vi "ELAPSED TIMER VI FOR Sway Loop Connection.vi"(8 "error in":errorcluster, 9 "TARGET":dbl, 10 "RESET":bool, 11 "PAUSE":bool) -> (0 "error out":errorcluster, 1 "ELAPSED INDICATION":bool, 2 "ELAPSED TIMER":dbl)   [LabVIEW 2025]
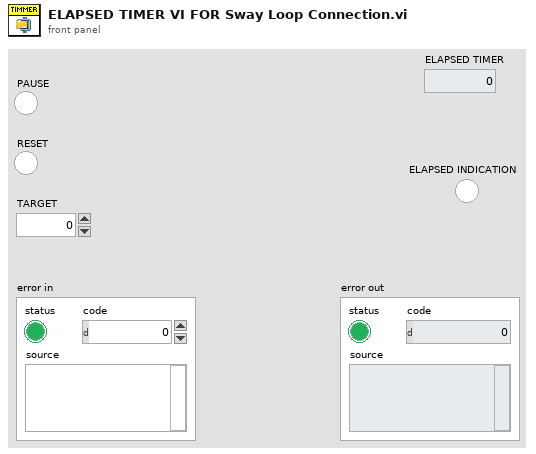
[diagram p1: front panel]
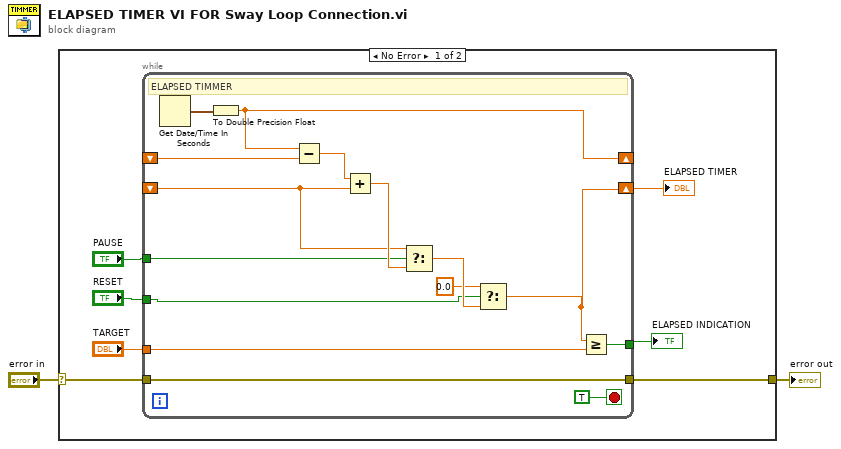
[diagram p0: block diagram]
diagram:
  n1 = case shown="No Error" "error in" {
    selector: "error in" -> [w4 _]
    tunnel: [w3 _] -> w1
    frame No Error {
      n2 = while {
        shift-right: [w21] -> _
        shift-left: _ -> [w22]
        shift-right: [w13] -> w6
        shift-left: _ -> [w18]
        tunnel: "PAUSE" -> [w17]
        tunnel: "RESET" -> [w14]
        tunnel: "TARGET" -> [w12]
        tunnel: [w11] -> w5
        tunnel: w4 -> [w10]
        tunnel: [w10] -> w3
        stop <- TRUE stop-if-true
        # "ELAPSED TIMMER"
        n3 = Get Date/Time In Seconds() -> (seconds since 1Jan1904=w23:timestamp)
        n4 = To Double Precision Float(number=w23) -> (double precision float=w21:dbl)
        n5 = Subtract(x=w21, y=w22) -> (x-y=w20:dbl)
        n6 = Add(x=w20, y=w18) -> (x+y=w19:dbl)
        n7 = Select(t=w18, s=w17, f=w19) -> (s? t:f=w16:dbl)
        n8 = Select(t=0.0, s=w14, f=w16) -> (s? t:f=w13:dbl)
        n9 = Greater Or Equal?(x=w13, y=w12) -> (x >= y?=w11:bool)
      }
      "ELAPSED TIMER" <- w6
      "ELAPSED INDICATION" <- w5
    }
    frame Error {
    }
  }
  "error out" <- w1
